vi "Read statement.vi"(8 "error in (no error)":errorcluster, 11 "LogStatementMsg in":refnum<class "LogStatementMsg.lvclass">) -> (0 "error out":errorcluster, 2 "Statement":T1={"timestamp"=timestamp(0 s since 1904-01-01), "level"=enum."INFO", "sourceTag"="", "originVI"="", "message"=""}, 3 "LogStatementMsg out":refnum<class "LogStatementMsg.lvclass">)   [LabVIEW 2026, in "Lumberjack.lvlib" / "LogStatementMsg.lvclass"]
uses:
  LogStatementMsg.lvclass
  TypeDefs/Statement.ctl
  TypeDefs/Severity.ctl
  LogStatementMsg.lvclass/LogStatementMsg.ctl
  Lumberjack.lvlib
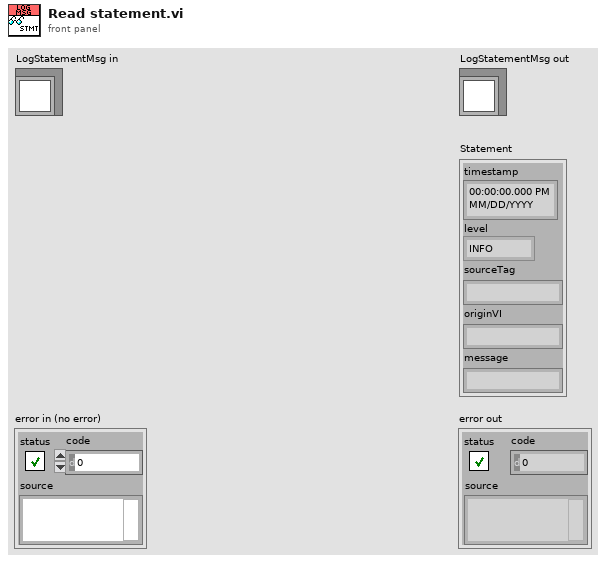
[diagram p1: front panel]
types:
  T1 = typedef "Lumberjack.lvlib/Statement.ctl" = cluster{"timestamp":timestamp, "level":T2, "sourceTag":string, "originVI":string, "message":string}
  T2 = typedef "Lumberjack.lvlib/Severity.ctl" = enum16{"OFF", "FATAL", "ERROR", "WARN", "INFO", "DEBUG", "TRACE", "ALL"}
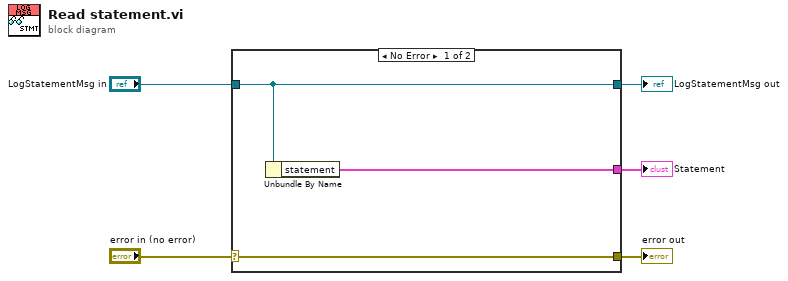
[diagram p0: block diagram]
diagram:
  n1 = case shown="No Error" "error in (no error)" {
    selector: "error in (no error)" -> [w8 w9]
    tunnel: [w8 w9] -> w4
    tunnel: [w7 w10] -> w2
    tunnel: "LogStatementMsg in" -> [w7 w10]
    tunnel: [w6 _] -> w1
    frame No Error {
      n2 = Unbundle By Name(w7) -> ("statement"=w6:T1)
    }
    frame Error {
    }
  }
  "error out" <- w4
  "LogStatementMsg out" <- w2
  "Statement" <- w1
